vi "TP_UI.vi"() -> ()   [LabVIEW 2012]
uses:
  controls/TP_UI Ref.ctl
  controls/TP_Privileges.ctl
panel:
  out "SN:":string
  out "Privileges:":string
  out "User:":string
  out "Test process Bar":u8(slide) scale=0.0..100.0
  in  "TRS":string(tree)
  in  "Info":enum32{"Message", "Error", "Toolbox"}(tab)
  out "Message":string
  out "Result":cluster{"TestResult":bool}
  out "Version:":string
  in  "SrciptList":string(combo)
  in  "error in":errorcluster
  in  "Test":bool
  in  "Stop":bool
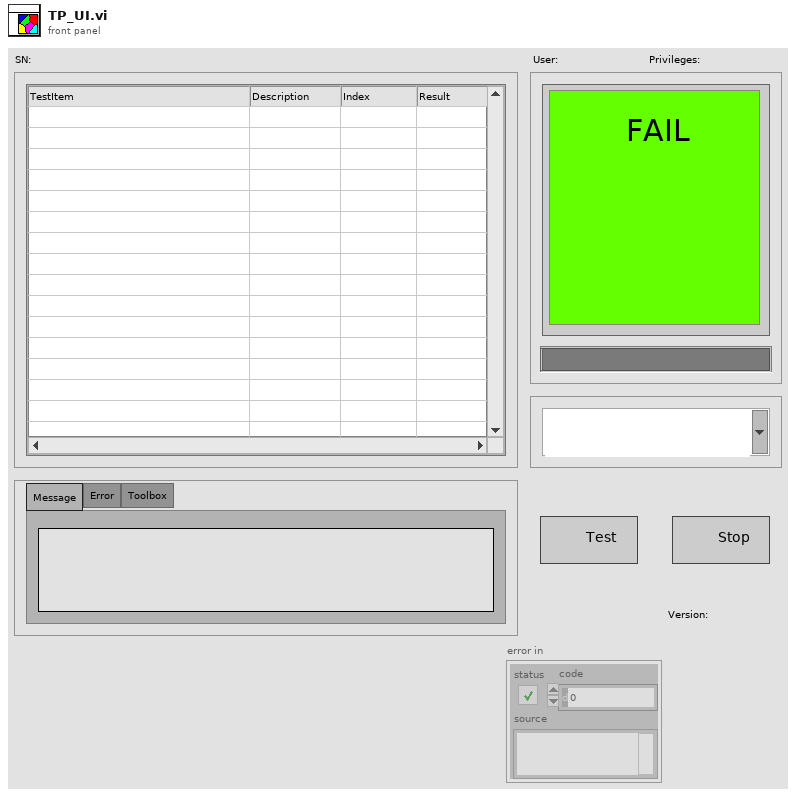
[diagram p1: front panel]
types:
  T1 = typedef "TP_Privileges.ctl" = enum16{"Anonymous", "User", "Debugger", "Developer", "Admin"}
  T2 = enum16{"Init", "GetValue", "SetValue", "Destory"}
  T3 = enum16{"Create Queue", "Get Queue", "Destory Queue", "Destory all Queue"}
  T4 = enum16{"Init", "GetValue", "SetValue", "Destory", "ErrLog"}
  T5 = typedef "TP_UI Ref.ctl" = cluster{"This VI":refnum<vi>, "String":refnum<vi>, "Test":refnum<vi>, "Quit":refnum<vi>, "SrciptList":refnum<vi>, "TRS":refnum<vi>, "Info":refnum<vi>, "Result":refnum<vi>, "menu":refnum<k9>}
  T6 = typedef "TP_Config.ctl" = cluster{"Info":cluster{"version":string, "date":string, "author":string, "mail":string}, "User_info":cluster{"username":string, "memery_enable":bool}, "Path":cluster{"script":string, "errlog":string}}
  T7 = cluster{"Config":T6, "UI_Ref":T5, "Privilege":T1, "Stop":bool}
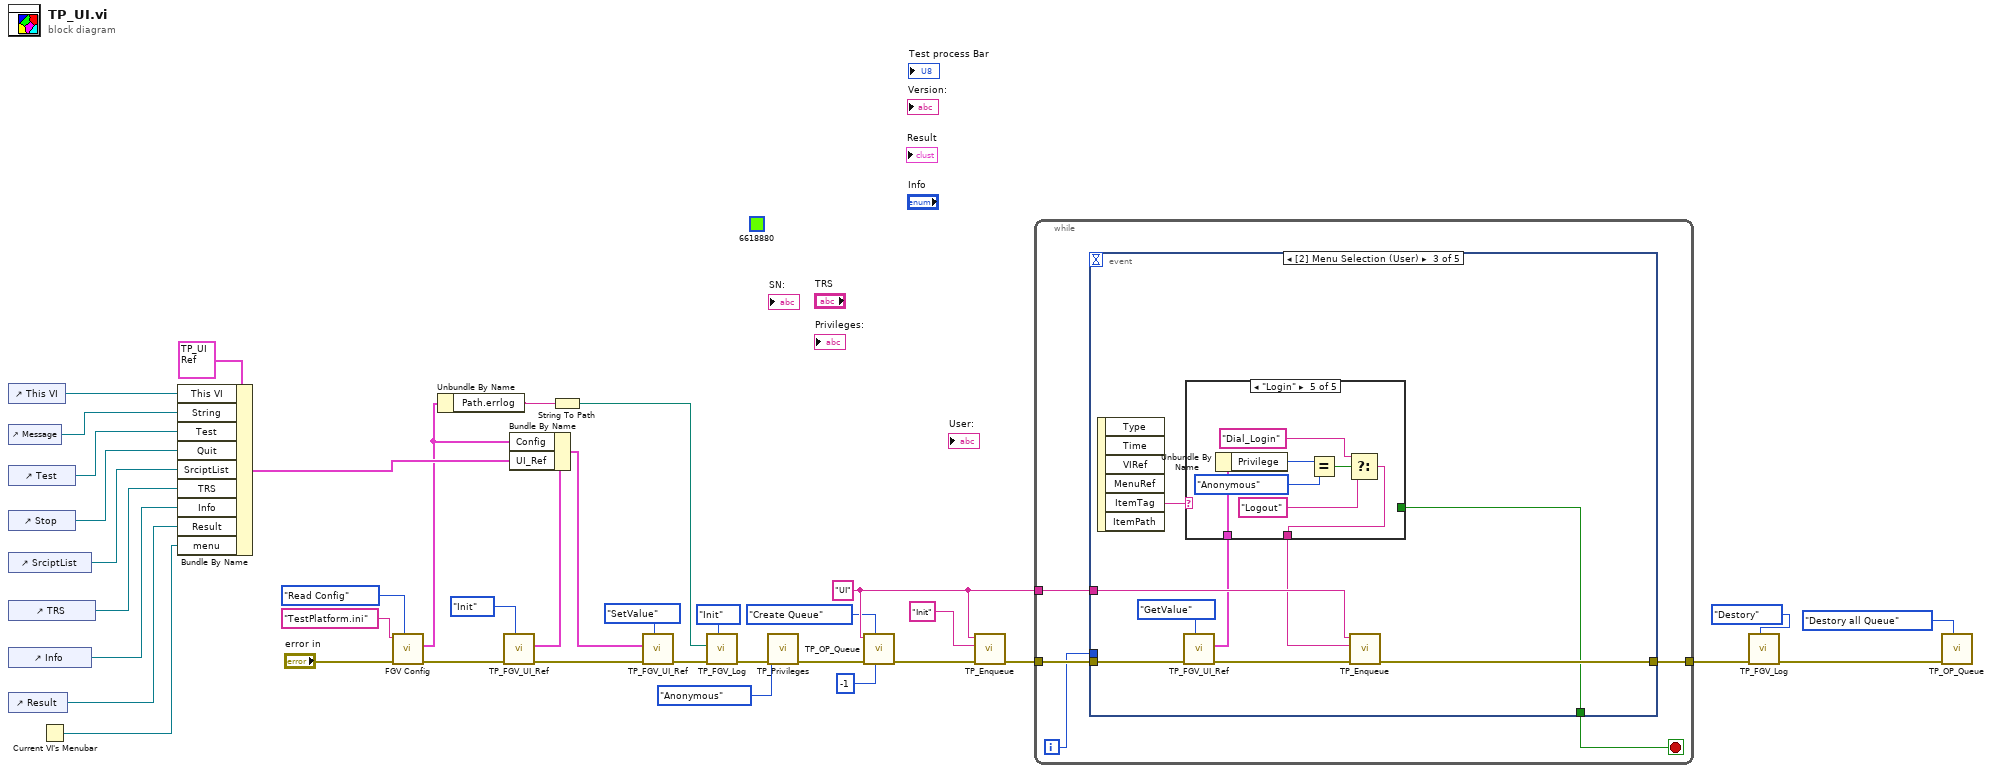
[diagram p0: block diagram]
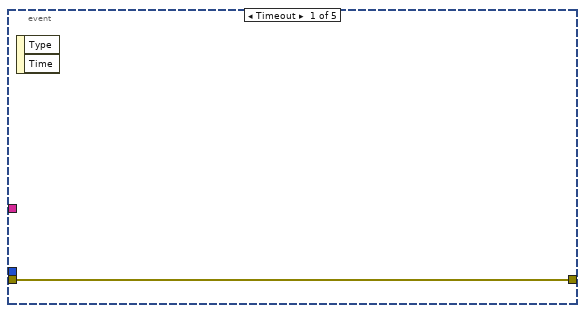
[diagram p2: hidden frame]
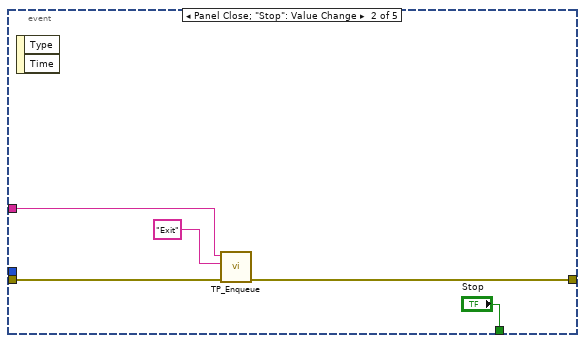
[diagram p3: hidden frame]
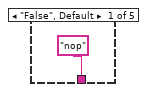
[diagram p4: hidden frame]
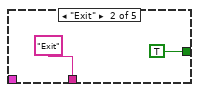
[diagram p5: hidden frame]
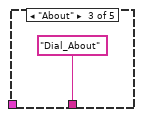
[diagram p6: hidden frame]
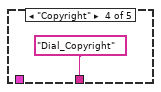
[diagram p7: hidden frame]
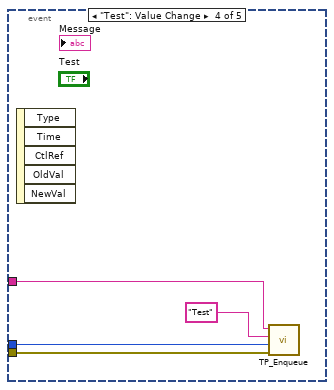
[diagram p8: hidden frame]
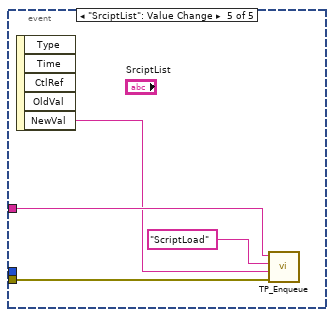
[diagram p9: hidden frame]
diagram:
  w23 = "UI" ("name (unnamed)")
  (unwired) u32 6618880 ("Color Box")
  n1 = control-ref of="This VI"() -> (w29:refnum<vi>)
  n2 = control-ref of="Message"() -> (w30:refnum<vi>)
  n3 = control-ref of="Test"() -> (w31:refnum<vi>)
  n4 = control-ref of="Stop"() -> (w32:refnum<vi>)
  n5 = control-ref of="SrciptList"() -> (w34:refnum<vi>)
  n6 = control-ref of="TRS"() -> (w33:refnum<vi>)
  n7 = control-ref of="Info"() -> (w35:refnum<vi>)
  n8 = control-ref of="Result"() -> (w36:refnum<vi>)
  n9 = Current VI's Menubar() -> (w4:refnum<k9>)
  n10 = Bundle By Name(cluster=T5 {"This VI"=refnum, "String"=refnum, "Test"=refnum, "Quit"=refnum, "SrciptList"=refnum, "TRS"=refnum, "Info"=refnum, "Result"=refnum, "menu"=refnum} ("UI_Ref out"), "This VI"=w29, "String"=w30, "Test"=w31, "Quit"=w32, "SrciptList"=w34, "TRS"=w33, "Info"=w35, "Result"=w36, "menu"=w4) -> (w14:T5)
  n11 = call "FGV Config.vi"("Enum"=enum16{"Read Config", "Save Config"}."Read Config", "error in"="error in", "config FName"="TestPlatform.ini") -> ("error out"=w10:errorcluster, "Config out"=w7:T6)  [unwired: 7 in]
  n12 = Unbundle By Name(w7) -> ("Path.errlog"=w6:string)
  n13 = call "TP_FGV_UI_Ref.vi"("Enum"=T2."Init", "error in (no error)"=w10) -> ("error out"=w12:errorcluster, "Global Variants out"=w15:T7)  [unwired: 8 in]
  n14 = Bundle By Name(cluster=w15, "Config"=w7, "UI_Ref"=w14) -> (w13:T7)
  n15 = String To Path(string=w6) -> (path=w5:path)
  n16 = call "TP_FGV_UI_Ref.vi"("Enum"=T2."SetValue", "error in (no error)"=w12, "Global Variants in"=w13) -> ("error out"=w22:errorcluster)  [unwired: 7 in, 1 out]
  n17 = call "TP_FGV_Log.vi"("Enum"=T4."Init", "error in"=w22, "Log Path"=w5) -> ("error out"=w3:errorcluster)  [unwired: 8 in]
  n18 = call "TP_Privileges.vi"("error in (no error)"=w3, "Privilege"=TP_Privileges."Anonymous") -> ("error out"=w2:errorcluster)  [unwired: 9 in]
  n19 = call "TP_OP_Queue.vi"("max queue size (-1, unlimited)"=-1, "OP_Queue (get queue)"=T3."Create Queue", "error in"=w2, "name (unnamed)"=w23) -> ("error out"=w24:errorcluster)  [unwired: 6 in, 1 out]
  n20 = call "TP_Enqueue.vi"("error in"=w24, "CMD"="Init", "name"=w23) -> ("error out"=w25:errorcluster)  [unwired: 8 in]
  n21 = while {
    tunnel: w25 -> [w43]
    tunnel: w23 -> [w41]
    tunnel: [w40] -> w20
    i -> [w42]
    stop <- w39 stop-if-true
    n22 = event shown="[2] Menu Selection (User)" {
      selector: _ -> [_ _ _ _ _]
      dyn-events: _ -> [_ _ _ _ _]
      timeout: _ -> [_ _ _ _ _]
      tunnel: w43 -> [w44 w48 w53 w74 w77]
      tunnel: [_ "Stop" w54 _ _] -> w39
      tunnel: w42 -> [_ _ _ w71 _]
      tunnel: w41 -> [_ w47 w57 w72 w76]
      tunnel: [w44 w45 w55 _ _] -> w40
      event Timeout {
        n23 = event-data() -> ()  [unwired: 1 in, 2 out]
      }
      event Panel Close; "Stop": Value Change {
        n24 = event-data() -> ()  [unwired: 1 in, 2 out]
        n25 = call "TP_Enqueue.vi"("error in"=w48, "CMD"="Exit", "name"=w47) -> ("error out"=w45:errorcluster)  [unwired: 8 in]
      }
      event Menu Selection (User) {
        n26 = event-data() -> ("ItemTag"=w58:string)  [unwired: 1 in, 5 out]
        n27 = call "TP_FGV_UI_Ref.vi"("Enum"=T2."GetValue", "error in (no error)"=w53) -> ("error out"=w52:errorcluster, "Global Variants out"=w51:T7)  [unwired: 8 in]
        n28 = case shown="\"Login\"" w58 {
          tunnel: ["nop" ("Message") "Exit" ("Message") "Dial_About" ("Message") "Dial_Copyright" ("Message") w66] -> w56
          tunnel: [_ TRUE _ _ _] -> w54
          tunnel: w51 -> [_ _ _ _ w70]
          frame "False", Default {
          }
          frame "Exit" {
          }
          frame "About" {
          }
          frame "Copyright" {
          }
          frame "Login" {
            n29 = Unbundle By Name(w70) -> ("Privilege"=w69:T1)
            n30 = Equal?(x=w69, y=TP_Privileges."Anonymous") -> (x = y?=w67:bool)
            n31 = Select(t="Dial_Login" ("Message"), s=w67, f="Logout") -> (s? t:f=w66:string)
          }
        }
        n32 = call "TP_Enqueue.vi"("error in"=w52, "CMD"=w56, "name"=w57) -> ("error out"=w55:errorcluster)  [unwired: 8 in]
      }
      event "Test": Value Change {
        n33 = event-data() -> ()  [unwired: 1 in, 5 out]
        n34 = call "TP_Enqueue.vi"("error in"=w74, "Paras"=w71, "CMD"="Test" ("Message"), "name"=w72) -> ()  [unwired: 7 in, 1 out]
      }
      event "SrciptList": Value Change {
        n35 = event-data() -> ("NewVal"=w75:string)  [unwired: 1 in, 4 out]
        n36 = call "TP_Enqueue.vi"("error in"=w77, "Paras"=w75, "CMD"="ScriptLoad" ("Message"), "name"=w76) -> ()  [unwired: 7 in, 1 out]
      }
    }
  }
  n37 = call "TP_FGV_Log.vi"("Enum"=T4."Destory", "error in"=w20) -> ("error out"=w19:errorcluster)  [unwired: 9 in]
  n38 = call "TP_OP_Queue.vi"("OP_Queue (get queue)"=T3."Destory all Queue", "error in"=w19) -> ()  [unwired: 8 in, 2 out]
